vi "GD_GWID11F_info.vi"(8 "error in (no error)":errorcluster, 9 "glue_id":string, 10 "evaluation_2":i16=1, 11 "DBlink":string="Driver={ODBC Driver 17 for SQL Server};Server=localhost\\SQLEXPRESS;Database=ZDX201;UID=labview;PWD=Dsa@54137926") -> (0 "error out":errorcluster)   [LabVIEW 2019]
uses:
  <vilib>/addons/database/Auxilliary.llb/DB Tools Format Datetime String (Time Stamp).vi
  <vilib>/addons/database/Connection.llb/DB Tools Open Connec (String).vi
  <vilib>/addons/database/NI_Database_API.lvlib
panel:
  out "Result":string
  out "Boolean array":bool[](array[boolean])
  out "Command 2":string="WHERE [id]=16"
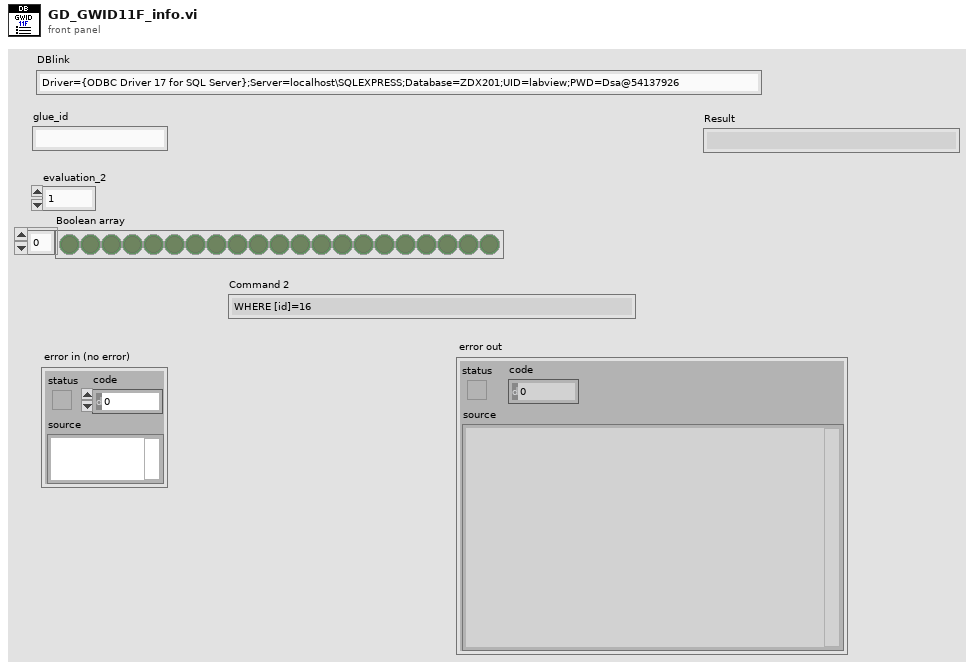
[diagram p1: front panel]
types:
  T1 = cluster{"evaluation_2":string, "update_time":timestamp, "eve_finish_2":timestamp}
  T2 = typedef "NI_Database_API.lvlib/Conn ObjectReference.ctl" = refnum<k1>
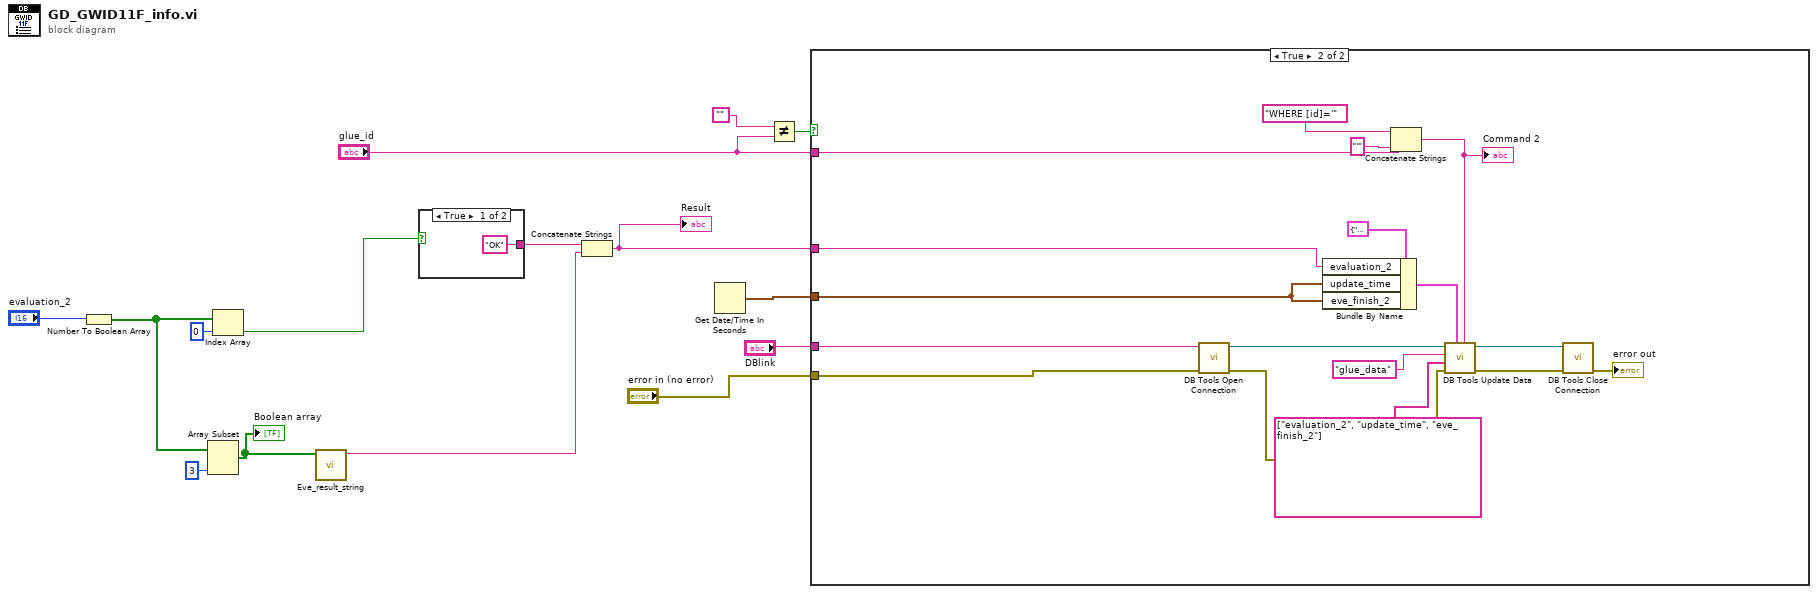
[diagram p0: block diagram]
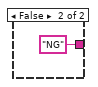
[diagram p2: hidden frame]
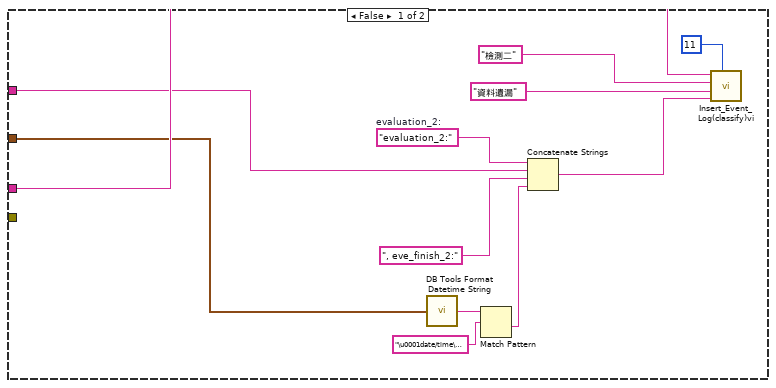
[diagram p3: hidden frame]
diagram:
  n1 = Number To Boolean Array(number="evaluation_2") -> (Boolean array=w3:bool[])
  n2 = Array Subset(array=w3, length=3) -> (w1:bool[])  [unwired: 1 in]
  "Boolean array" <- w1
  n3 = Index Array(array=w3, index=0) -> (element=w8:bool)
  n4 = call "Eve_result_string.vi"("Boolean array"=w1) -> ("String"=w5:string)  [unwired: 10 in]
  n5 = case shown="True" w8 {
    tunnel: ["OK" "NG"] -> w6
    frame True {
    }
    frame False {
    }
  }
  n6 = Concatenate Strings(w6, w5) -> (w4:string)
  "Result" <- w4
  n7 = Get Date/Time In Seconds() -> (seconds since 1Jan1904=w15:timestamp)
  n8 = Not Equal?(x="", y="glue_id") -> (x != y?=w12:bool)
  n9 = case shown="True" w12 {
    tunnel: w15 -> [w19 w37]
    tunnel: "DBlink" -> [w20 w33]
    tunnel: "error in (no error)" -> [_ w32]
    tunnel: "glue_id" -> [_ w31]
    tunnel: w4 -> [w18 w30]
    frame False {
      w21 = "evaluation_2:"  # evaluation_2:
      n10 = call-poly <vilib>:"DB Tools Format Datetime String.vi"("time stamp"=w19) -> ("date/time string"=w26:string)
      n11 = Match Pattern(string=w26, regular expression="\u0001date/time\u0001" ("search string")) -> (after substring=w24:string)  [unwired: 1 in, 3 out]
      n12 = Concatenate Strings(w21, w18, ", eve_finish_2:", w24) -> (w23:string)
      n13 = call "Insert_Event_Log(classify)vi.vi"("classify"=i16 11, "data"=w23, "message"="資料遺漏", "id"="檢測二", "DBlink"=w20) -> ()  [unwired: 6 in, 1 out]
    }
    frame True {
      n14 = call-poly <vilib>:"DB Tools Open Connection.vi"("error in (no error)"=w32, "connection information"=w33) -> ("error out"=w45:errorcluster, "connection reference"=w38:T2)  [unwired: 6 in]
      n15 = Bundle By Name(cluster=T1 {"evaluation_2"="", "update_time"=timestamp(0 s since 1904-01-01), "eve_finish_2"=timestamp(0 s since 1904-01-01)}, "evaluation_2"=w30, "update_time"=w37, "eve_finish_2"=w37) -> (w39:T1)
      n16 = Concatenate Strings("WHERE [id]='", w31, "'" ("string")) -> (w34:string)
      "Command 2" <- w34
      n17 = call <vilib>:"DB Tools Update Data.vi"("condition"=w34, "data"=w39, "error in (no error)"=w45, "columns"=string[] ["evaluation_2", "update_time", "eve_finish_2"], "table"="glue_data", "connection reference"=w38) -> ("error out"=w46:errorcluster, "connection reference out"=w44:T2)  [unwired: 4 in]
      n18 = call <vilib>:"DB Tools Close Connection.vi"("error in (no error)"=w46, "connection reference"=w44) -> ("error out"=→"error out":errorcluster)  [unwired: 5 in]
    }
  }
